vi "Get Scalar Datatypes and Refs.vi"(8 "error in (no error)":errorcluster, 10 "Item GUID":string, 11 "Section Ref in":T5 format="%.0x") -> (0 "error out":errorcluster, 1 "Default Values":dbl[](array[numeric]), 2 "VS Ref":T5[](array[typedef]) format="%.0x", 3 "Section Ref out":T5 format="%.0x", 4 "Registers Ref":T1[](array[typedef]) {"Register"."Data Type" format="%.0x"})   [LabVIEW 2016, in "FPGA Addon System Explorer.lvlib"]
uses:
  FPGA Addon System Explorer.lvlib
  <vilib>/NI Veristand/Custom Device API/Custom Device Item Ref.ctl
  Shared/Compiled.RegisterSettings.ctl
  Shared/Scalar Type.ctl
  Shared/Register Information.ctl
  Shared/Data Type.ctl
  <vilib>/NI Veristand/Custom Device API/Get Item Property (String).vi
  convert RegisterMap to FPGA Scalar.vi
  Get Controls RegisterMap.vi
  VeriStand-FPGA-Resource-Manager/Source/find Relative VS Ref.vi
  Get Indicators RegisterMap.vi
  <vilib>/NI Veristand/Custom Device Tools/Custom Device Utility Library/NI VeriStand - Search for Item by GUID.vi
  Shared/Constants.vi
  <vilib>/NI VeriStand/Custom Device API/Custom Device API.lvlib
  <vilib>/NI VeriStand/Custom Device Tools/Custom Device Utility Library/Custom Device Utility Library.lvlib
  Shared/FPGA Addon Shared.lvlib
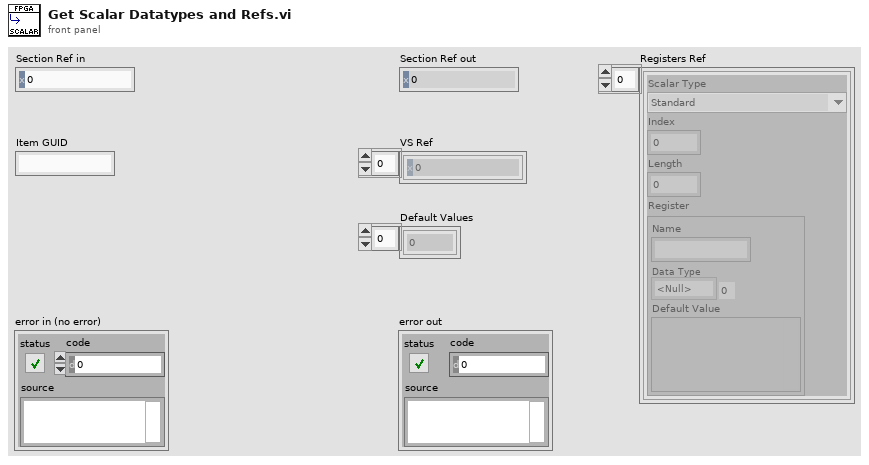
[diagram p1: front panel]
types:
  T1 = typedef "FPGA Addon Shared.lvlib/Compiled.RegisterSettings.ctl" = cluster{"Scalar Type":T2, "Index":i32, "Length":i32, "Register":T3}
  T2 = typedef "FPGA Addon Shared.lvlib/Scalar Type.ctl" = enum16{"Standard", "Bitpacked"}
  T3 = typedef "FPGA Addon Shared.lvlib/Register Information.ctl" = cluster{"Name":string, "Data Type":T4, "Default Value":variant}
  T4 = typedef "FPGA Addon Shared.lvlib/Data Type.ctl" = enum8{"<Null>", "I8", "I16", "I32", "I64", "U8", "U16", "U32", "U64", "SGL", "Boolean", "Analog PWM In Settings", "Analog PWM In", "Digital PWM In Settings", "Digital PWM In", "Digital PWM Out", "Sine Out", "FXP+/-24.5", "FXP+/-16.5", "FXP+/-32.8", "FXP+/-64.32", "FXP+/-16.7", "FXP+/-20.5"}
  T5 = typedef "Custom Device API.lvlib/Custom Device Item Ref.ctl" = u64
  T6 = typedef "Custom Device API.lvlib/Custom Device Item Info.ctl" = cluster{"Name":string, "Is Channel":bool, "GUID":string, "Is Waveform":bool}
  T7 = typedef "Custom Device API.lvlib/Custom Device Channel.ctl" = cluster{"Type":T8, "Units":string, "Default Value":dbl, "Faultable":bool, "Scalable":bool}
  T8 = typedef "Custom Device API.lvlib/Custom Device Channel Type.ctl" = enum16{"Input", "Output"}
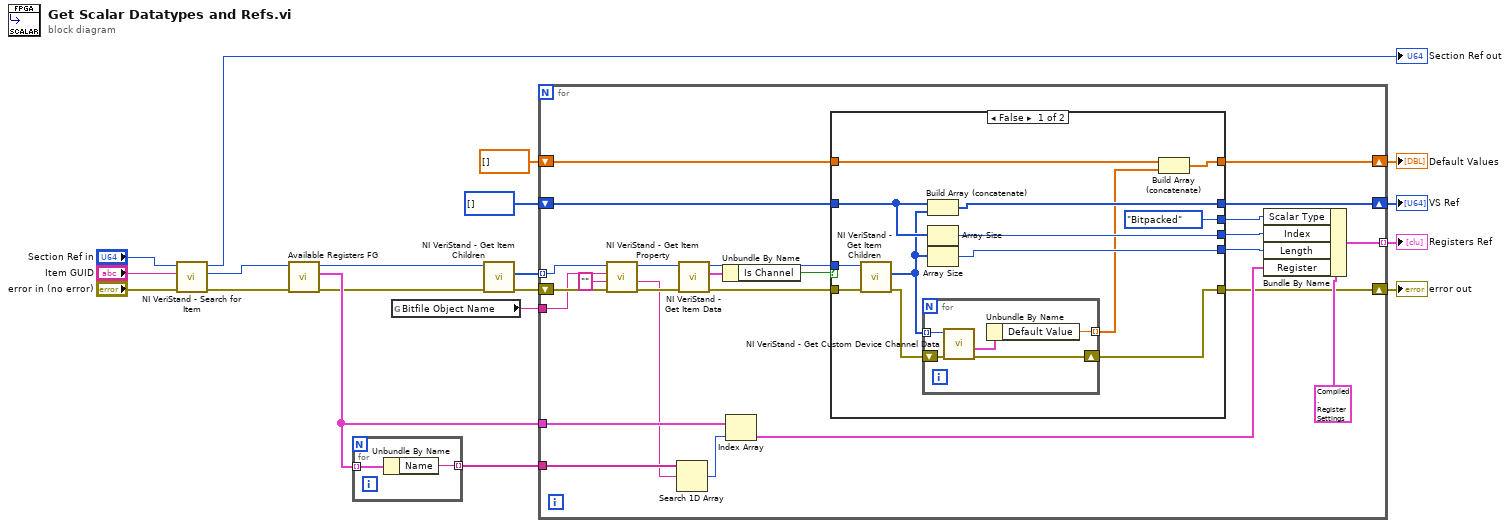
[diagram p0: block diagram]
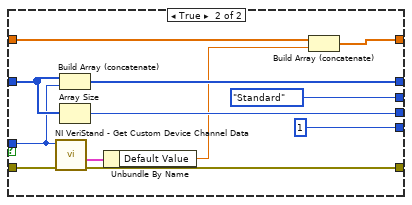
[diagram p2: hidden frame]
diagram:
  n1 = call-poly <vilib>:"NI VeriStand - Search for Item.vi"("error in"="error in (no error)", "Item GUID"="Item GUID", "Section Ref in"="Section Ref in") -> ("error out"=w18:errorcluster, "Item Ref"=w19:T5, "Section Ref out"=→"Section Ref out":T5)  [unwired: 5 in, 1 out]
  n2 = call "Available Registers FG.vi"("error in (no error)"=w18, "Item Ref"=w19) -> ("error out"=w15:errorcluster, "Available Registers"=w16:T3[], "Item Ref out"=w17:T5)  [unwired: 7 in]
  n3 = for {
    tunnel: w16 -> [w21] mode=indexing
    tunnel: [w20] -> w14 mode=indexing
    n4 = Unbundle By Name(w21) -> ("Name"=w20:string)
  }
  n5 = global read "Constants.vi" "Bitfile Object Name"() -> (w13:string)
  n6 = call <vilib>:"NI VeriStand - Get Item Children.vi"("error in (no error)"=w15, "Item Ref in"=w17) -> ("error out"=w11:errorcluster, "Child Refs"=w12:T5[])  [unwired: 6 in, 2 out]
  n7 = for {
    shift-right: [w24] -> w6
    shift-left: w11 -> [w46]
    tunnel: w12 -> [w45] mode=indexing
    tunnel: w13 -> [w44]
    tunnel: w14 -> [w42]
    tunnel: w16 -> [w40]
    shift-right: [w32] -> w4
    shift-left: T5[] [] -> [w33]
    tunnel: [w31] -> w5 mode=indexing
    shift-right: [w23] -> w1
    shift-left: dbl[] [] -> [w22]
    n8 = call-poly <vilib>:"NI VeriStand - Get Item Property.vi"("error in (no error)"=w46, "Default Value"="", "Property Name"=w44, "Item Ref in"=w45) -> ("error out"=w38:errorcluster, "Value"=w30:string, "Item Ref out"=w41:T5)  [unwired: 4 in, 1 out]
    n9 = Search 1D Array(1D array=w42, element=w30) -> (index of element=w39:i32)  [unwired: 1 in]
    n10 = call <vilib>:"NI VeriStand - Get Item Data.vi"("error in (no error)"=w38, "Item Ref in"=w41) -> ("error out"=w35:errorcluster, "Item Info"=w37:T6, "Item Ref out"=w36:T5)  [unwired: 6 in, 1 out]
    n11 = Unbundle By Name(w37) -> ("Is Channel"=w34:bool)
    n12 = Index Array(array=w40, index=w39) -> (element=w25:T3)
    n13 = case shown="False" w34 {
      tunnel: w36 -> [w58 w71]
      tunnel: w35 -> [w59 w70]
      tunnel: [w49 w69] -> w24
      tunnel: w33 -> [w56 w74]
      tunnel: [w57 w76] -> w32
      tunnel: [Scalar_Type."Bitpacked" ("Scalar Type") Scalar_Type."Standard" ("Scalar Type")] -> w29
      tunnel: [w55 w73] -> w28
      tunnel: [w54 1] -> w27
      tunnel: [w47 w66] -> w23
      tunnel: w22 -> [w51 w65]
      frame False {
        n14 = call <vilib>:"NI VeriStand - Get Item Children.vi"("error in (no error)"=w59, "Item Ref in"=w58) -> ("error out"=w50:errorcluster, "Child Refs"=w52:T5[])  [unwired: 6 in, 2 out]
        n15 = for {
          tunnel: w52 -> [w63] mode=indexing
          shift-right: [w61] -> w49
          shift-left: w50 -> [w62]
          tunnel: [w60] -> w48 mode=indexing
          n16 = call <vilib>:"NI VeriStand - Get Custom Device Channel Data.vi"("error in (no error)"=w62, "Channel Ref in"=w63) -> ("error out"=w61:errorcluster, "Channel"=w64:T7)  [unwired: 4 in, 4 out]
          n17 = Unbundle By Name(w64) -> ("Default Value"=w60:dbl)
        }
        n18 = Build Array (concatenate)(w56, w52) -> (w57:T5[])
        n19 = Array Size(array=w56) -> (size(s)=w55:i32)
        n20 = Array Size(array=w52) -> (size(s)=w54:i32)
        n21 = Build Array (concatenate)(w51, w48) -> (w47:dbl[])
      }
      frame True {
        n22 = call <vilib>:"NI VeriStand - Get Custom Device Channel Data.vi"("error in (no error)"=w70, "Channel Ref in"=w71) -> ("error out"=w69:errorcluster, "Channel"=w68:T7)  [unwired: 4 in, 4 out]
        n23 = Build Array (concatenate)(w74, w71) -> (w76:T5[])
        n24 = Array Size(array=w74) -> (size(s)=w73:i32)
        n25 = Unbundle By Name(w68) -> ("Default Value"=w67:dbl)
        n26 = Build Array (concatenate)(w65, w67) -> (w66:dbl[])
      }
    }
    n27 = Bundle By Name(cluster=T1 {"Scalar Type"=enum."Standard", "Index"=0, "Length"=0, "Register"={"Name"="", "Data Type"=enum."<Null>", "Default Value"=variant(dbl 0.0)}} ("Cluster"), "Scalar Type"=w29, "Index"=w28, "Length"=w27, "Register"=w25) -> (w31:T1)
  }
  "error out" <- w6
  "VS Ref" <- w4
  "Registers Ref" <- w5
  "Default Values" <- w1
